vi "Array2Matrix.vi"(1 "Array":sgl[](array[numeric]), 2 "Header":string[](array[string])) -> (0 "Array2D":sgl[][](array[numeric]))   [LabVIEW 2021]
panel:
  out "size(s)":i32[](array[numeric])
  out "Array3":sgl[](array[numeric])
  # "Columns are the number of signals\nRows are the length of each signal"
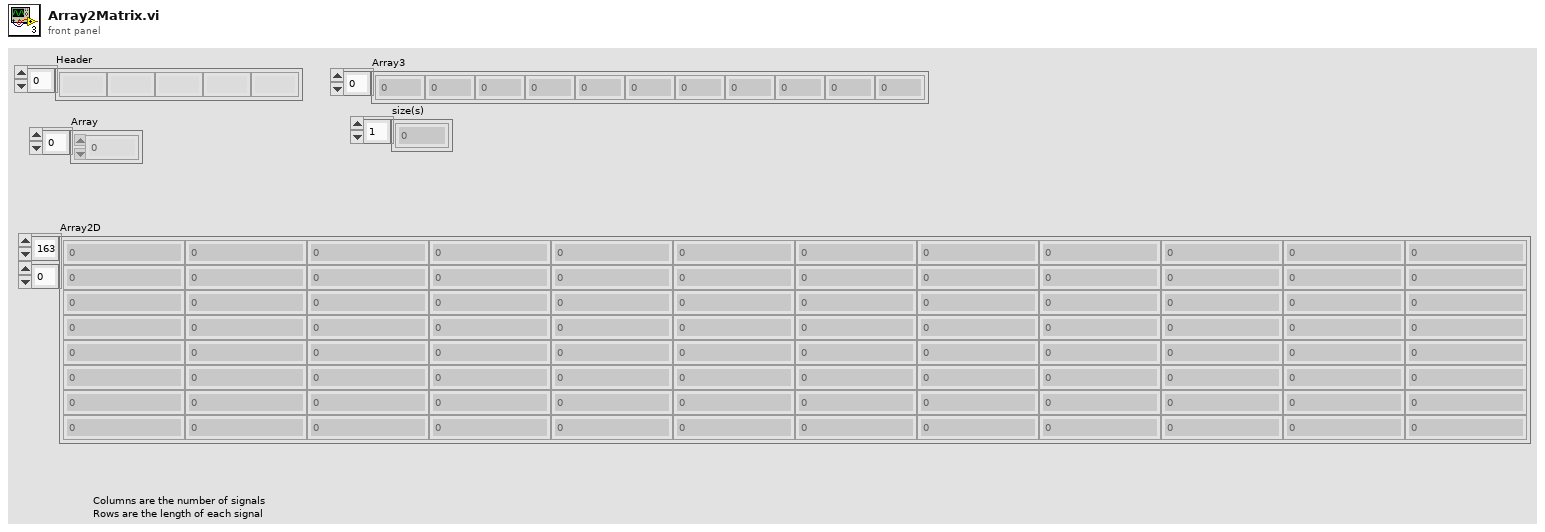
[diagram p1: front panel]
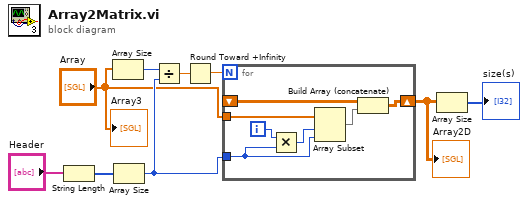
[diagram p0: block diagram]
diagram:
  n1 = String Length(string="Header") -> (length=w8:i32[])
  n2 = Array Size(array="Array") -> (size(s)=w2:i32)
  n3 = Array Size(array=w8) -> (size(s)=w7:i32)
  n4 = Divide(x=w2, y=w7) -> (x/y=w9:dbl)
  n5 = Round Toward +Infinity(x=w9) -> (ceil(x): smallest int >= x=w6:dbl)
  n6 = for {
    N: w6 -> [_]
    tunnel: "Array" -> [w16]
    tunnel: w7 -> [w10]
    shift-right: [w15] -> w3
    shift-left: _ -> [w13]
    i -> [w12]
    n7 = Multiply(x=w12, y=w10) -> (x*y=w11:i32)
    n8 = Array Subset(array=w16, index=w11, length=w10) -> (w14:sgl[])
    n9 = Build Array (concatenate)(w13, w14) -> (w15:sgl[][])
  }
  "Array2D" <- w3
  n10 = Array Size(array=w3) -> (size(s)=→"size(s)":i32[])
  "Array3" <- "Array"
